vi "Simple.vi"() -> ()   [LabVIEW 2023]
panel:
  out "Boolean":bool
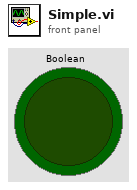
[diagram p1: front panel]
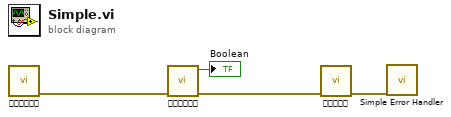
[diagram p0: block diagram]
diagram:
  n1 = call "설정.vi"() -> ("error out"=w4:errorcluster)  [unwired: 11 in]
  n2 = call "측정.vi"("error in"=w4) -> ("error out"=w3:errorcluster, "Boolean"=→"Boolean":bool)  [unwired: 9 in]
  n3 = call "종료.vi"("error in"=w3) -> ("error out"=w2:errorcluster)  [unwired: 10 in]
  n4 = call <vilib>:"Simple Error Handler.vi"("error in (no error)"=w2) -> ()  [unwired: 4 in, 5 out]
